vi "Reference Enqueue Message (Array).vi"(6 "Priority Message? Array":bool[](array[boolean]), 7 "Queue":string, 8 "error in":errorcluster, 9 "Message Data Array":variant[](array[variant]), 10 "Message Array":string[](array[string]), 11 "VI Ref":refnum<vi>) -> (0 "error out":errorcluster)   [LabVIEW 2021, in "Message Queue.lvlib"]
doc: "Obtains a Reference ot the Queue and then enqueues an array of messages/data. \nFor a regular message, enqueue the message. For a priority message, enqueue it at the front of the queue."
uses:
  Message Queue.lvlib
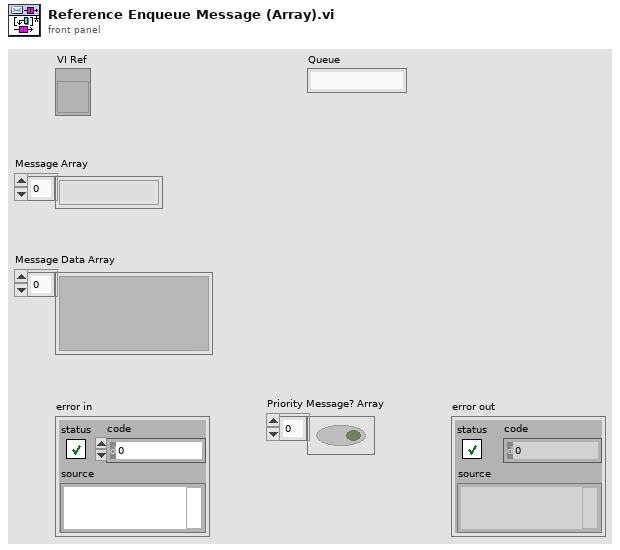
[diagram p1: front panel]
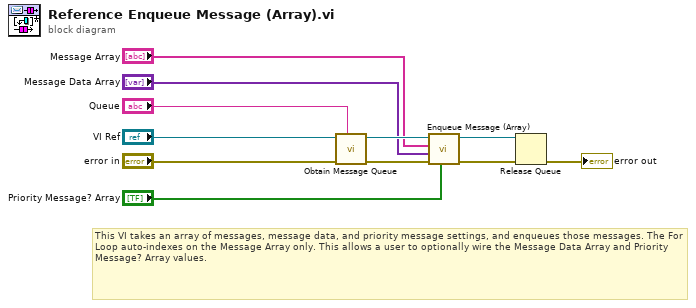
[diagram p0: block diagram]
diagram:
  # "This VI takes an array of messages, message data, and priority message settings, and enqueues those messages. The For Loop auto-indexes on the Message Array only. This allows a user to optionally wire the Message Data Array and Priority Message? Array values."
  n1 = call "Obtain Message Queue.vi"("Queue"="Queue", "error in"="error in", "VI Ref"="VI Ref") -> ("error out"=w11:errorcluster, "Message Queue"=w7:refnum<queue>)  [unwired: 7 in]
  n2 = call "Enqueue Message (Array).vi"("Priority Message? Array"="Priority Message? Array", "error in (no error)"=w11, "Message Data Array"="Message Data Array", "Message Array"="Message Array", "Message Queue"=w7) -> ("error out"=w3:errorcluster, "dup Message Queue"=w1:refnum<queue>)  [unwired: 5 in]
  n3 = Release Queue(queue=w1, error in (no error)=w3) -> (error out=→"error out":errorcluster)  [unwired: 1 in, 2 out]
